vi "From JSON.vi"(8 "error in (no error)":errorcluster, 10 "JSON":string, 11 "Double Float in":refnum<class "Abs_Extended Float.lvclass">) -> (0 "error out":errorcluster, 3 "Double Float out":refnum<class "Abs_Extended Float.lvclass">)   [LabVIEW 2021, in "Abs_Extended Float.lvclass"]
uses:
  Abs_Extended Float.lvclass
  C:/Program Files (x86)/National Instruments/LabVIEW 2021/vi.lib/TSA/Abstract Data Classes/Abs_Types/Type/Abs_Type.lvclass
  Support/Type.ctl
  46d3848b-86a9-4f9c-9358-c1b5147e4345.vi
  <vilib>/JDP Science/JSONtext/Find Item.vi
  <vilib>/JDP Science/JSONtext/Next JSON Value.vi
  <vilib>/JDP Science/JSONtext/String Subset.vi
  <vilib>/JDP Science/JSONtext/Parsing/Advance past next JSON Value (inlined COPY).vi
  <vilib>/JDP Science/JSONtext/Parsing/Advance past whitespace.vi
  <vilib>/JDP Science/JSONtext/Parsing/Advance past String.vi
  <vilib>/JDP Science/JSONtext/Parsing/Advance past Number.vi
  <vilib>/JDP Science/JSONtext/Parsing/Advance past Line Ending.vi
  <vilib>/Utility/LVClass/Get LV Class Name.vi
  <vilib>/JDP Science/JSONtext/Parsing/Parse Full Path or Item Name.vi
  <vilib>/JDP Science/JSONtext/Parsing/Advance past Array.vi
  <vilib>/JDP Science/JSONtext/Parsing/Advance past Object.vi
  <vilib>/JDP Science/JSONtext/support/Error Cluster From Code.vi
  <vilib>/JDP Science/JSONtext/Offset/Find Item Locations by Path.vi
  <vilib>/JDP Science/JSONtext/JSON text to Variant.vi
  Type/Abs_Type.lvclass
  <vilib>/JDP Science/JSONtext/LVClass Serializer/JSONtext LVClass Serializer.lvclass
  Floating Point/Abs_Floating Point.lvclass
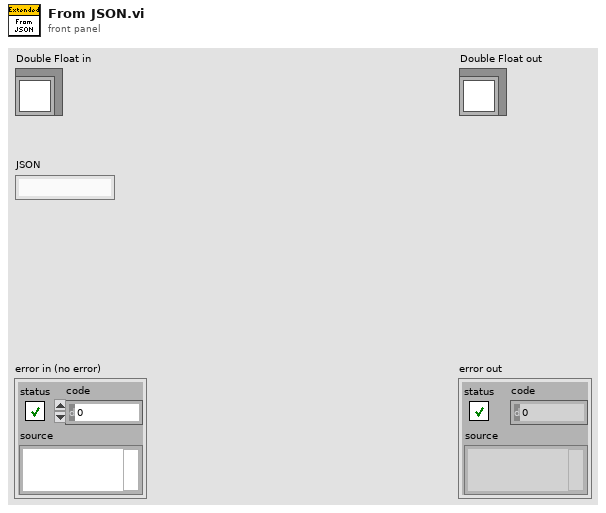
[diagram p1: front panel]
types:
  T1 = typedef "Abs_Extended Float.lvclass/Type.ctl" = ext
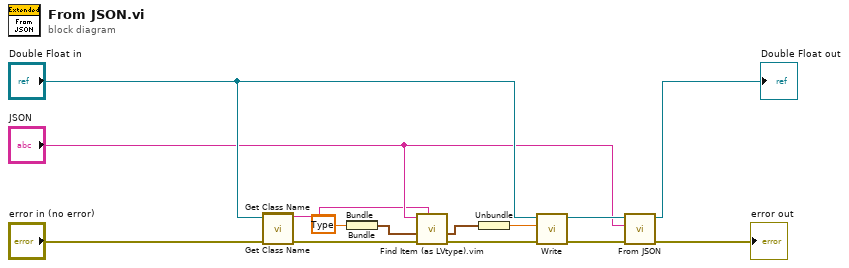
[diagram p0: block diagram]
diagram:
  n1 = call "Get Class Name.vi"() -> ("class name"=w1:string)  [unwired: 10 in, 1 out]
  n2 = call "Get Class Name.vi"("error in (no error)"="error in (no error)", "Abs_Type in"="Double Float in") -> ("error out"=w2:errorcluster)  [unwired: 8 in, 1 out]
  n3 = Bundle("Value"=T1 0.0) -> ()  [unwired: 1 in, 1 out]
  n4 = Bundle("Value"=T1 0.0) -> (w10:cluster{"Value":T1})  [unwired: 1 in]
  n5 = call "Find Item (as LVtype).vim"("$Path or Item Name"=w1, "error in (no error)"=w2, "Data Type and Default Value"=w10, "JSON"="JSON") -> ("error out"=w9:errorcluster, "Data"=w11:cluster{"Value":T1})  [unwired: 4 in, 2 out]
  n6 = Unbundle(w11) -> ("Value"=w6:T1)
  n7 = call-dynamic "Write.vi"("error in (no error)"=w9, "Value"=w6, "Double Float.lvclass_340760 in"="Double Float in") -> ("error out"=w8:errorcluster, "Double Float.lvclass_340760 out"=w7:refnum<class "Abs_Extended Float.lvclass">)  [unwired: 7 in]
  n8 = call-parent "From JSON.vi"("error in (no error)"=w8, "JSON"="JSON", "Type in"=w7) -> ("error out"=→"error out":errorcluster, "Type out"=→"Double Float out":refnum<class "Abs_Extended Float.lvclass">)  [unwired: 7 in]
